vi "Interpolation (with Init Mem) Test.vi"() -> ()   [LabVIEW 2014]
uses:
  <vilib>/FPGAPlugInAG/sbRIO-9636/niLvFpga_Open_sbRIO-9636.vi
  <vilib>/rvi/interface/common/dynamic/niFpgaDynamicAddResources.vi
  <vilib>/rvi/interface/common/niFpgaWaitOnOcc.vi
  <vilib>/Utility/error.llb/Error Cluster From Error Code.vi
  <vilib>/FPGAPlugInAG/Dynamic/niLvFpga_Reset_Dynamic.vi
  <vilib>/FPGAPlugInAG/Dynamic/niLvFpga_Run_Dynamic.vi
  <vilib>/rvi/errors/niLvFpgaAdjustHostInterfaceError.vi
  <vilib>/RVI Host/nirviSupport.llb/nirviErrorClusterFromErrorCode.vi
  <vilib>/FPGAPlugInAG/Dynamic/niLvFpga_Abort_Dynamic.vi
  <vilib>/FPGAPlugInAG/Dynamic/niLvFpga_Close_Dynamic.vi
  <vilib>/rvi/interface/nirviOpenFPGA/nirviOpenFPGA.xnode
  FPGA Bitfiles/LaserDistanceSen_FPGATarget_DoubleFFTMesuram_eAomBu3ZaMU.lvbitx
  FPGA Target/Test VIs/Double FFT Mesurament (Max Bin detection & Init Mem) test.vi
  <vilib>/rvi/interface/nirviMethod/nirviMethod.xnode
  <vilib>/rvi/interface/nirviCloseFPGA/nirviCloseFPGA.xnode
  <vilib>/FPGAPlugInAG/Dynamic/niLvFpga_ConfigureFifo_Dynamic.vi
  <vilib>/rvi/errors/niLvFpgaMergeErrorWithErrorCode.vi
  <vilib>/FPGAPlugInAG/Dynamic/niLvFpga_StartFifo_Dynamic.vi
  <vilib>/rvi/interface/nirviMethod/StockFPGA_InlinedMethodWaitForSingleIRQ.vi
  <vilib>/FPGAPlugInAG/Dynamic/niLvFpga_WaitOnIrq_Dynamic.vi
  <vilib>/FPGAPlugInAG/Dynamic/niLvFpga_AcknowledgeIrq_Dynamic.vi
  <vilib>/FPGAPlugInAG/Dynamic/niLvFpga_WriteFifo_Dynamic.vi
panel:
  out "Detected Frequency (Hz)":dbl
  in  "stop":bool
  out "Max Bin":i32
  out "Max Amp":dbl format="%.2f"
  out "Prev Bin":i32
  out "Next Bin":i32
  out "Prev Amp":dbl format="%.2f"
  out "Next Amp":dbl format="%.2f"
  out "Interpolated Bin":dbl
  in  "Interpolation Method":T1(ring)
  out "Write Memory Complete":bool
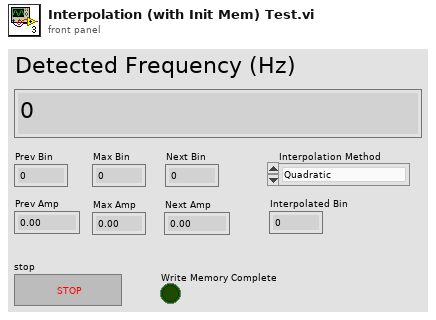
[diagram p1: front panel]
types:
  T1 = enum16{"Quadratic", "McLeodd", "Barycentric", "Jain"}
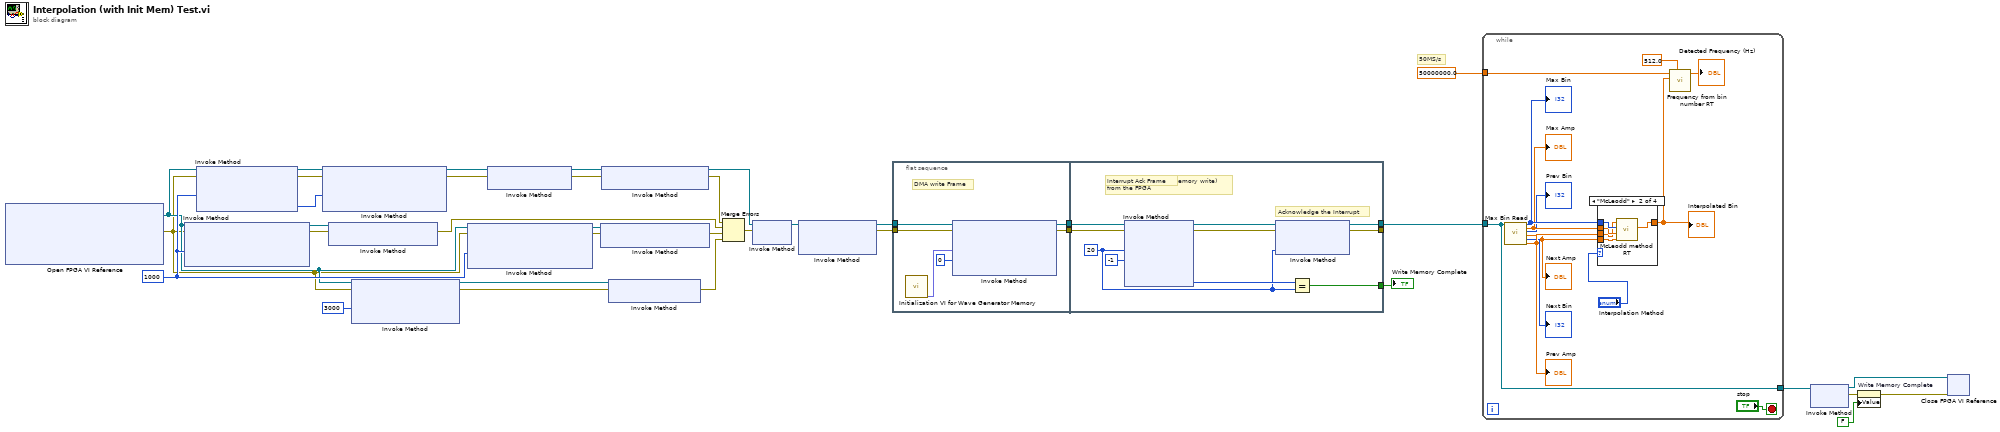
[diagram p0: block diagram]
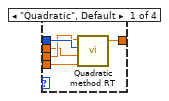
[diagram p2: hidden frame]
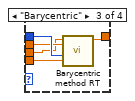
[diagram p3: hidden frame]
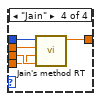
[diagram p4: hidden frame]
diagram:
  w24 = u32 1000 ("Requested Depth")
  # "50MS/s"
  n1 = xnode "Open FPGA VI Reference"() -> ("FPGA VI Reference Out"=w19:refnum<k20>, "error out"=w18:errorcluster)  [unwired: 2 in]
  n2 = xnode "Invoke Method"("FPGA VI Reference In"=w19, "error in"=w18, "Requested Depth"=w24) -> ("FPGA VI Reference Out"=w25:refnum<k20>, "error out"=w26:errorcluster)  [unwired: 1 out]
  n3 = xnode "Invoke Method"("FPGA VI Reference In"=w19, "error in"=w18, "Requested Depth"=w24) -> ("FPGA VI Reference Out"=w36:refnum<k20>, "error out"=w35:errorcluster, "Actual Depth"=w34:u32)
  n4 = xnode "Invoke Method"("FPGA VI Reference In"=w36, "error in"=w35, "Requested Depth"=w34) -> ("FPGA VI Reference Out"=w33:refnum<k20>, "error out"=w32:errorcluster)  [unwired: 1 out]
  n5 = xnode "Invoke Method"("FPGA VI Reference In"=w25, "error in"=w26) -> ("error out"=w28:errorcluster)  [unwired: 1 out]
  n6 = xnode "Invoke Method"("FPGA VI Reference In"=w19, "error in"=w18, "Requested Depth"=u32 3000) -> ("FPGA VI Reference Out"=w21:refnum<k20>, "error out"=w20:errorcluster)  [unwired: 1 out]
  n7 = xnode "Invoke Method"("FPGA VI Reference In"=w19, "error in"=w18, "Requested Depth"=w24) -> ("FPGA VI Reference Out"=w23:refnum<k20>, "error out"=w22:errorcluster)  [unwired: 1 out]
  n8 = xnode "Invoke Method"("FPGA VI Reference In"=w33, "error in"=w32) -> ("FPGA VI Reference Out"=w31:refnum<k20>, "error out"=w30:errorcluster)
  n9 = xnode "Invoke Method"("FPGA VI Reference In"=w23, "error in"=w22) -> ("error out"=w27:errorcluster)  [unwired: 1 out]
  n10 = xnode "Invoke Method"("FPGA VI Reference In"=w31, "error in"=w30) -> ("FPGA VI Reference Out"=w13:refnum<k20>, "error out"=w29:errorcluster)
  n11 = xnode "Invoke Method"("FPGA VI Reference In"=w21, "error in"=w20) -> ("error out"=w16:errorcluster)  [unwired: 1 out]
  n12 = Merge Errors(w29, w28, w27, w16) -> (w14:errorcluster)
  n13 = xnode "Invoke Method"("FPGA VI Reference In"=w13, "error in"=w14) -> ("FPGA VI Reference Out"=w15:refnum<k20>)  [unwired: 1 out]
  n14 = xnode "Invoke Method"("FPGA VI Reference In"=w15) -> ("FPGA VI Reference Out"=w10:refnum<k20>, "error out"=w9:errorcluster)  [unwired: 2 in]
  n15 = flat-sequence {
    tunnel: [w41] -> w12
    tunnel: [w40] -> w11
    tunnel: w10 -> [w38]
    tunnel: w9 -> [w37]
    tunnel: [w46] -> w4
    tunnel: [w47] -> _
    tunnel: w12 -> [w51]
    tunnel: w11 -> [w52]
    tunnel: [w43] -> w8
    frame #0 {
      # "DMA write Frame"
      n16 = call "Initialization VI for Wave Generator Memory.vi"() -> ("FXP Init Data Out"=w39:fxp<+/-,12,12>[])  [unwired: 10 in, 1 out]
      n17 = xnode "Invoke Method"("FPGA VI Reference In"=w38, "error in"=w37, "Data"=w39, "Timeout (ms)"=0) -> ("FPGA VI Reference Out"=w41:refnum<k20>, "error out"=w40:errorcluster)  [unwired: 1 out]
    }
    frame #1 {
      w44 = 20 ("IRQ Number(s)")
      # "Acknowledge the Interrupt"
      # "Wait for interrupt 20 (Memory write)\nfrom the FPGA"
      # "Interrupt Ack Frame"
      n18 = xnode "Invoke Method"("FPGA VI Reference In"=w51, "error in"=w52, "IRQ Number(s)"=w44, "Timeout (ms)"=-1) -> ("FPGA VI Reference Out"=w48:refnum<k20>, "error out"=w49:errorcluster, "IRQ(s) Asserted"=w45:i32)  [unwired: 1 out]
      n19 = xnode "Invoke Method"("FPGA VI Reference In"=w48, "error in"=w49, "IRQ Number(s)"=w44) -> ("FPGA VI Reference Out"=w46:refnum<k20>, "error out"=w47:errorcluster)
      n20 = Equal?(x=w45, y=w44) -> (x = y?=w43:bool)
    }
  }
  n21 = while {
    tunnel: w4 -> [w57]
    tunnel: 50000000.0 ("Sample Rate (S/s)") -> [w60]
    tunnel: [w57] -> w5
    stop <- "stop" stop-if-true
    n22 = call "Max Bin Read.vi"("FPGA VI Reference In"=w57) -> ("Max Bin"=w65:i32, "Max Amp"=w64:dbl, "Prev Bin"=→"Prev Bin":i32, "Next Amp"=w58:dbl, "Next Bin"=→"Next Bin":i32, "Prev Amp"=w59:dbl)  [unwired: 13 in]
    "Max Bin" <- w65
    "Max Amp" <- w64
    "Prev Amp" <- w59
    "Next Amp" <- w58
    n23 = case shown="\"McLeodd\"" "Interpolation Method" {
      tunnel: w65 -> [w69 w74 w79 w84]
      tunnel: w64 -> [w66 w73 w78 w83]
      tunnel: w59 -> [w67 w72 w77 w82]
      tunnel: w58 -> [w68 w71 w76 w81]
      tunnel: [w70 w75 w80 w85] -> w54
      frame "Quadratic", Default {
        n24 = call "Quadratic method RT.vi"("Next Amplitude"=w68, "Max Amplitude"=w66, "Max bin"=w69, "Prev Amplitude"=w67) -> ("Bin"=w70:dbl)  [unwired: 7 in]
      }
      frame "McLeodd" {
        n25 = call "McLeodd method RT.vi"("Next Amp"=w71, "Max Amp"=w73, "Max Bin"=w74, "Prev Amp"=w72) -> ("Bin"=w75:dbl)  [unwired: 7 in]
      }
      frame "Barycentric" {
        n26 = call "Barycentric method RT.vi"("Next Amp"=w76, "Max Bin"=w79, "Max Amp"=w78, "Prev Amp"=w77) -> ("Bin"=w80:dbl)  [unwired: 7 in]
      }
      frame "Jain" {
        n27 = call "Jain's method RT.vi"("Prev Amp"=w82, "Next Amp"=w81, "Max Amp"=w83, "Max Bin"=w84) -> ("Bin"=w85:dbl)  [unwired: 7 in]
      }
    }
    "Interpolated Bin" <- w54
    n28 = call "Frequency from bin number RT.vi"("FFT size"=512.0, "Bin number"=w54, "Sample Rate (S/s)"=w60) -> ("Detected Frequency (Hz)"=→"Detected Frequency (Hz)":dbl)  [unwired: 8 in]
  }
  n29 = xnode "Invoke Method"("FPGA VI Reference In"=w5) -> ("FPGA VI Reference Out"=w6:refnum<k20>, "error out"=w3:errorcluster)  [unwired: 1 in]
  n30 = property on="Write Memory Complete" class="Bool (strict)"(error in=w3, "Value"=FALSE ("Write Memory Complete")) -> (error out=w2:errorcluster)  [unwired: 1 in, 1 out]
  n31 = xnode "Close FPGA VI Reference"("FPGA VI Reference In"=w6, "error in"=w2) -> ()  [unwired: 1 out]
  "Write Memory Complete" <- w8
